vi "Post-Build Action.vi"(5 "Files Generated by Build":path[](array[path]), 6 "Top Level/Always Included VIs":path[](array[path]), 7 "Destination Path":path, 8 "error in (no error)":errorcluster, 9 "Target Name":string, 10 "Build Specification Name":string, 11 "Project Path":path) -> (0 "error out":errorcluster)   [LabVIEW 2014]
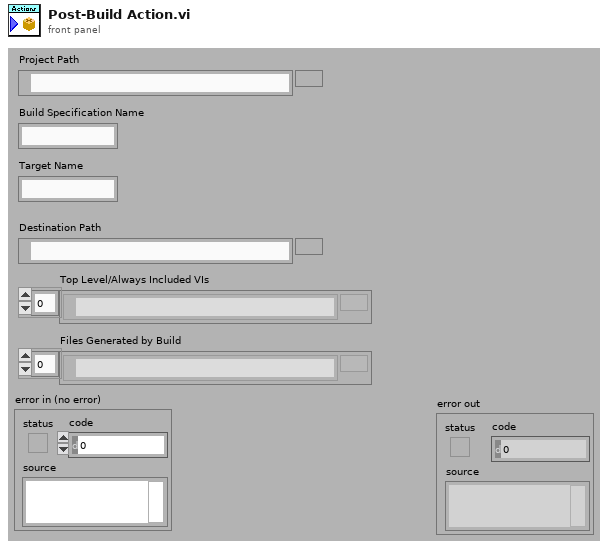
[diagram p1: front panel]
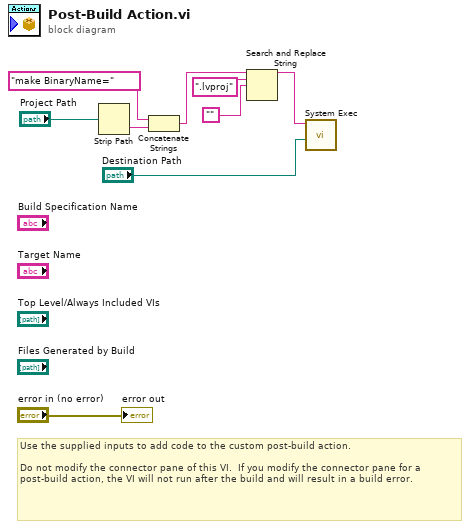
[diagram p0: block diagram]
diagram:
  # "Use the supplied inputs to add code to the custom post-build action.\n\nDo not modify the connector pane of this VI.  If you modify the connector pane for a post-build action, the VI will not run after the build and will result in a build error."
  n1 = Strip Path(path="Project Path") -> (name=w5:string)  [unwired: 1 out]
  n2 = Concatenate Strings("make BinaryName=" ("command line"), w5) -> (w4:string)
  n3 = Search and Replace String(input string=w4, search string=".lvproj", replace string="") -> (result string=w3:string)  [unwired: 5 in, 3 out]
  n4 = call <vilib>:"System Exec.vi"("working directory"="Destination Path", "command line"=w3) -> ()  [unwired: 6 in, 4 out]
  "error out" <- "error in (no error)"
